vi "remindUserViIsRunning.vi"(8 "error in":errorcluster, 9 "enumIndex":i32, 10 "Enum Refnum":refnum<vi>, 11 "VI reference in":refnum<vi>) -> (0 "error out":errorcluster, 3 "VI reference out":refnum<vi>)   [LabVIEW 2010]
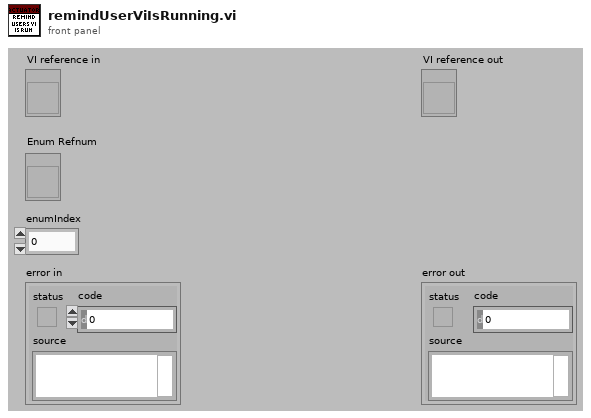
[diagram p1: front panel]
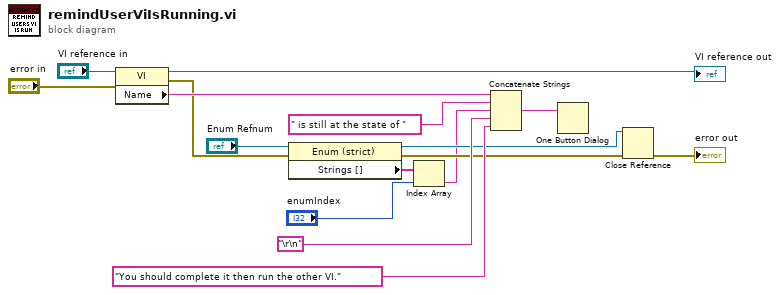
[diagram p0: block diagram]
diagram:
  n1 = property class="VI"(reference="VI reference in", error in="error in") -> (reference out=→"VI reference out":refnum<vi>, error out=w8:errorcluster, "Name"=w15:string)
  n2 = property on="Property Node" class="Enum (strict)"(reference="Enum Refnum", error in=w8) -> (reference out=w6:refnum<vi>, error out=w7:errorcluster, "Strings []"=w3:string[])
  n3 = Index Array(array=w3, index="enumIndex") -> (element=w1:string)
  n4 = Concatenate Strings(w15, " is still at the state of ", w1, "\r\n", "You should complete it then run the other VI.") -> (w12:string)
  n5 = One Button Dialog(message=w12) -> ()  [unwired: 1 in, 1 out]
  n6 = Close Reference(reference=w6, error in (no error)=w7) -> (error out=→"error out":errorcluster)
